vi "Profile_UpdateGUI.vi"(9 "Data Cluster":T1, 10 "Configuration Cluster":T3={"General"={"Config.ini"=path "", "Default Logging Path"=path ""}, "Hardware"={"AHC VISA COM"="", "Measure Rate (1/s)"=0, "Global T VAR"="", "Global B VAR"=""}, "Operation"={"Operation Mode"=enum."Idle-Off", "Status"="", "NewLog?"=FALSE}}) -> (1 "Data Cluster Out":T1, 2 "Configuration Cluster Out":T3={"General"={"Config.ini"=path "", "Default Logging Path"=path ""}, "Hardware"={"AHC VISA COM"="", "Measure Rate (1/s)"=0, "Global T VAR"="", "Global B VAR"=""}, "Operation"={"Operation Mode"=enum."Idle-Off", "Status"="", "NewLog?"=FALSE}})   [LabVIEW 2021]
uses:
  Config_Cluster.ctl
  Data_Cluster.ctl
  Mode_Enum.ctl
  Measurement_Cluster.ctl
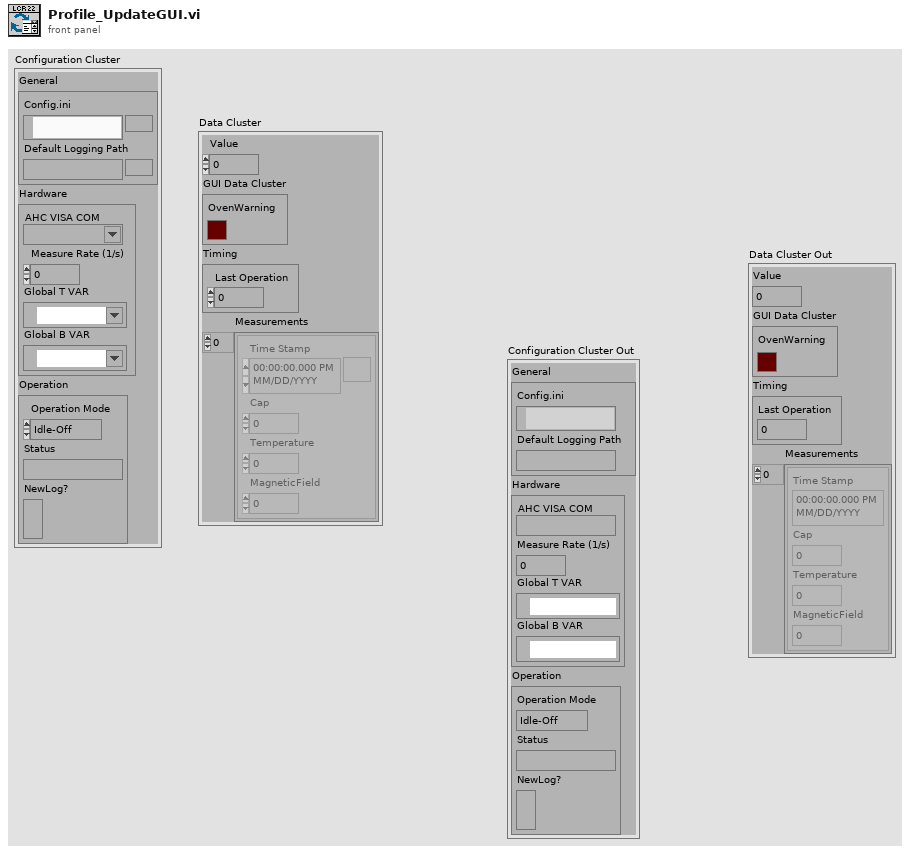
[diagram p1: front panel]
types:
  T1 = typedef "Data_Cluster.ctl" = cluster{"Value":dbl, "GUI Data Cluster":cluster{"OvenWarning":bool}, "Timing":cluster{"Last Operation":dbl}, "Measurements":T2[]}
  T2 = typedef "Measurement_Cluster.ctl" = cluster{"Time Stamp":timestamp, "Cap":dbl, "Temperature":dbl, "MagneticField":dbl}
  T3 = typedef "Config_Cluster.ctl" = cluster{"General":cluster{"Config.ini":path, "Default Logging Path":path}, "Hardware":cluster{"AHC VISA COM":refnum<visa-resource-name>, "Measure Rate (1/s)":i32, "Global T VAR":refnum<k21>, "Global B VAR":refnum<k21>}, "Operation":cluster{"Operation Mode":T4, "Status":string, "NewLog?":bool}}
  T4 = typedef "Mode_Enum.ctl" = enum16{"Logging", "Idle-Off", "Idle"}
  T5 = cluster{"Bias Profile":cluster{" Bias Source (OFF)":u8, " Bias Type (Voltage)":u8, "Bias Level (0)":dbl}, "Measurement Profile":cluster{"Operation Mode (0: Auto)":u16, "Circuit Type (2: Auto)":u16, "Manual Range (1:Range 1 and 25 Ohms)":u8, "Auto Range (T: Enable)":bool}, "Signal Profile":cluster{"Frequency (1kHz)":dbl, "Measuring Voltage (1V)":dbl}, "Integration Profile":cluster{"Averaging (0: Off)":u16, "Averaging Number (2)":i32, "Time (100ms)":i32, "Rate (0: Fast)":u16}, "Trigger Profile":cluster{"Trigger Mode (0: Continuous)":u16}}
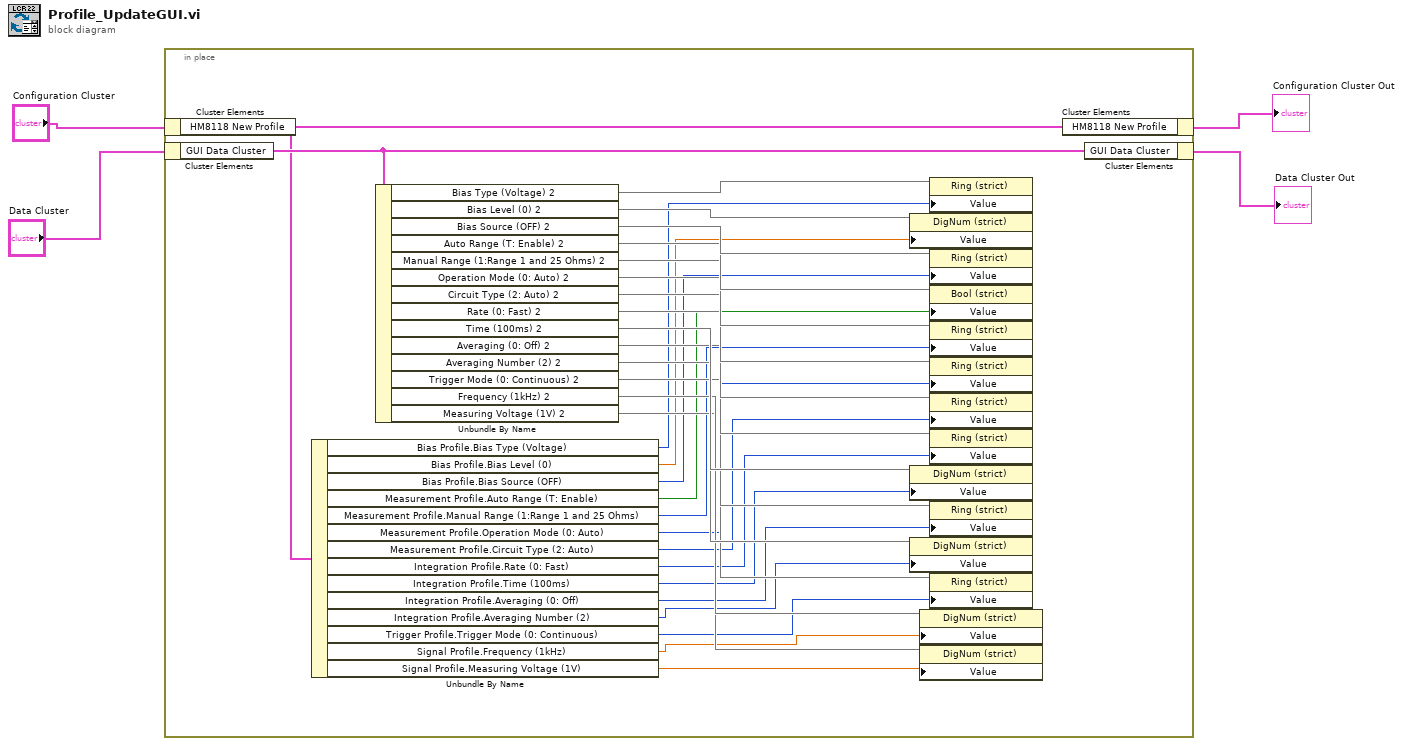
[diagram p0: block diagram]
diagram:
  n1 = in-place {
    n2 = in-place-cluster #1("Configuration Cluster") -> ("HM8118 New Profile"=w33:T5)
    n3 = in-place-cluster #2("Data Cluster") -> ("GUI Data Cluster"=w34:cluster{"OvenWarning":bool})
    n4 = Unbundle By Name(w33) -> ("Bias Profile.Bias Type (Voltage)"=w18:u8, "Bias Profile.Bias Level (0)"=w17:dbl, "Bias Profile.Bias Source (OFF)"=w16:u8, "Measurement Profile.Auto Range (T: Enable)"=w15:bool, "Measurement Profile.Manual Range (1:Range 1 and 25 Ohms)"=w14:u8, "Measurement Profile.Operation Mode (0: Auto)"=w13:u16, "Measurement Profile.Circuit Type (2: Auto)"=w12:u16, "Integration Profile.Rate (0: Fast)"=w11:u16, "Integration Profile.Time (100ms)"=w10:i32, "Integration Profile.Averaging (0: Off)"=w9:u16, "Integration Profile.Averaging Number (2)"=w8:i32, "Trigger Profile.Trigger Mode (0: Continuous)"=w7:u16, "Signal Profile.Frequency (1kHz)"=w6:dbl, "Signal Profile.Measuring Voltage (1V)"=w5:dbl)
    n5 = Unbundle By Name(w34) -> ("Bias Type (Voltage) 2"=w32, "Bias Level (0) 2"=w31, "Bias Source (OFF) 2"=w30, "Auto Range (T: Enable) 2"=w29, "Manual Range (1:Range 1 and 25 Ohms) 2"=w28, "Operation Mode (0: Auto) 2"=w27, "Circuit Type (2: Auto) 2"=w26, "Rate (0: Fast) 2"=w25, "Time (100ms) 2"=w24, "Averaging (0: Off) 2"=w23, "Averaging Number (2) 2"=w22, "Trigger Mode (0: Continuous) 2"=w21, "Frequency (1kHz) 2"=w20, "Measuring Voltage (1V) 2"=w19)
    n6 = property class="DigNum (strict)"(reference=w31, "Value"=w17) -> ()  [unwired: 1 in, 2 out]
    n7 = property class="DigNum (strict)"(reference=w24, "Value"=w10) -> ()  [unwired: 1 in, 2 out]
    n8 = property class="DigNum (strict)"(reference=w22, "Value"=w8) -> ()  [unwired: 1 in, 2 out]
    n9 = property class="DigNum (strict)"(reference=w20, "Value"=w6) -> ()  [unwired: 1 in, 2 out]
    n10 = property class="DigNum (strict)"(reference=w19, "Value"=w5) -> ()  [unwired: 1 in, 2 out]
    n11 = property class="Ring (strict)"(reference=w32, "Value"=w18) -> ()  [unwired: 1 in, 2 out]
    n12 = property class="Ring (strict)"(reference=w30, "Value"=w16) -> ()  [unwired: 1 in, 2 out]
    n13 = property class="Bool (strict)"(reference=w29, "Value"=w15) -> ()  [unwired: 1 in, 2 out]
    n14 = property class="Ring (strict)"(reference=w28, "Value"=w14) -> ()  [unwired: 1 in, 2 out]
    n15 = property class="Ring (strict)"(reference=w27, "Value"=w13) -> ()  [unwired: 1 in, 2 out]
    n16 = property class="Ring (strict)"(reference=w26, "Value"=w12) -> ()  [unwired: 1 in, 2 out]
    n17 = property class="Ring (strict)"(reference=w25, "Value"=w11) -> ()  [unwired: 1 in, 2 out]
    n18 = property class="Ring (strict)"(reference=w23, "Value"=w9) -> ()  [unwired: 1 in, 2 out]
    n19 = property class="Ring (strict)"(reference=w21, "Value"=w7) -> ()  [unwired: 1 in, 2 out]
    n20 = in-place-cluster #1("HM8118 New Profile"=w33) -> (→"Configuration Cluster Out":T3)
    n21 = in-place-cluster #2("GUI Data Cluster"=w34) -> (→"Data Cluster Out":T1)
  }
